vi "Autonomous Independent.vi"   [LabVIEW 2015]
doc: "This VI is called when autonomous begins, and will automatically be terminated when autonomous ends. You can carry out timed or sensor driven robot movement independently without needing to return to the caller."
uses:
  <vilib>/Rock Robotics/WPI/Utilities/WPI_GetSetVariantRefNum.vi
  <vilib>/Rock Robotics/Network Tables/NT Read String.vi
  <vilib>/Rock Robotics/Network Tables/NT Read Number.vi
  <vilib>/Rock Robotics/Network Tables/NT Read Boolean.vi
  <vilib>/Rock Robotics/Network Tables/NT Write Numeric Array.vi
panel:
  # "Be sure to right-click and choose Data Operations>>Make Current Value default if you want to save the array values with the VI"
types:
  T1 = typedef "WPI_JoystickDevRef.ctl" = cluster{"Device":T2}
  T2 = typedef "WPI_JoystickDeviceEnum.ctl" = enum16{"USB 0", "USB 1", "USB 2", "USB 3", "USB 4", "USB 5"}
  T3 = typedef "WPI_EncoderDevRef.ctl" = cluster{"DevStatus":errorcluster, "EncoderIndex":T4, "CounterIndex":T5, "DistancePerCount":dbl, "Decoding Type":T6}
  T4 = typedef "FPGA_EncoderIdx.ctl" = enum8{"Enc 0", "Enc 1", "Enc 2", "Enc 3", "Enc 4", "Enc 5", "Enc 6", "Enc 7", "Invalid"}
  T5 = typedef "FPGA_CounterCtrSystemIndex.ctl" = enum8{"Ctr 0", "Ctr 1", "Ctr 2", "Ctr 3", "Ctr 4", "Ctr 5", "Ctr 6", "Ctr 7", "Invalid"}
  T6 = typedef "WPI_EncoderType.ctl" = enum16{"1x", "2x", "4x"}
  T7 = typedef "WPI_GyroDevRef.ctl" = cluster{"DevStatus":errorcluster, "Analog Channel":T8, "Offset":dbl, "Gain (VoltsPerDegree/Second)":dbl, "Gyro Type":enum16{"Analog", "XRS450"}, "Handle":i32, "SPI Bus":T9, "Device Found":bool, "Sample Rate":dbl, "Calibrate On Open":bool}
  T8 = typedef "FPGA_AIChannel.ctl" = enum8{"AI 0", "AI 1", "AI 2", "AI 3", "AI MXP 0", "AI MXP 1", "AI MXP 2", "AI MXP 3", "Invalid"}
  T9 = typedef "spi_bus.ctl" = enum16{"SPI On-Board, CS0", "SPI On-Board, CS1", "SPI On-Board, CS2", "SPI On-Board, CS3", "SPI MXP", "Invalid"}
  T10 = typedef "WPI_RobotDriveDevRef.ctl" = cluster{"DevStatus":errorcluster, "Motors[]":T11[], "Square Inputs":bool, "Max Output":dbl}
  T11 = typedef "WPI_MotorControlDeviceRef.ctl" = cluster{"DeviceStatus":errorcluster, "Type":T12, "PWM":cluster{"PWM Channel":T13, "DeadBand":T14}, "CAN":cluster{"Device Number":u8, "Control Mode":T15, "Semaphore":T16, "Max Vout":dbl, "TalonSRX Control Mode":T17}, "Invert":bool}
  T12 = typedef "WPI_MotorControlType.ctl" = enum16{"PWM", "CAN", "CANTalonSRX"}
  T13 = typedef "FPGA_DIOPWMChannel.ctl" = enum8{"PWM 0", "PWM 1", "PWM 2", "PWM 3", "PWM 4", "PWM 5", "PWM 6", "PWM 7", "PWM 8", "PWM 9", "PWM MXP 0", "PWM MXP 1", "PWM MXP 2", "PWM MXP 3", "PWM MXP 4", "PWM MXP 5", "PWM MXP 6", "PWM MXP 7", "PWM MXP 8", "PWM MXP 9", "Invalid"}
  T14 = typedef "WPI_PWMDeadband.ctl" = cluster{"Name":string, "maxPositivePwm":i32, "minPositivePwm":i32, "centerPwm":i32, "maxNegativePwm":i32, "minNegativePwm":i32, "angularRange":u16}
  T15 = typedef "WPI_CANJaguar_ControlMode.ctl" = enum8{"Percent VBus", "Current", "Speed", "Position", "Voltage"}
  T16 = typedef "Semaphore RefNum" = refnum<k1>
  T17 = typedef "WPI_CANTalonSRX_APIControlMode.ctl" = enum8{"Percent VBus", "Speed", "Position", "Slave", "Unchanged / Invalid", "Voltage Compensation", "Current", "Motion Profile"}
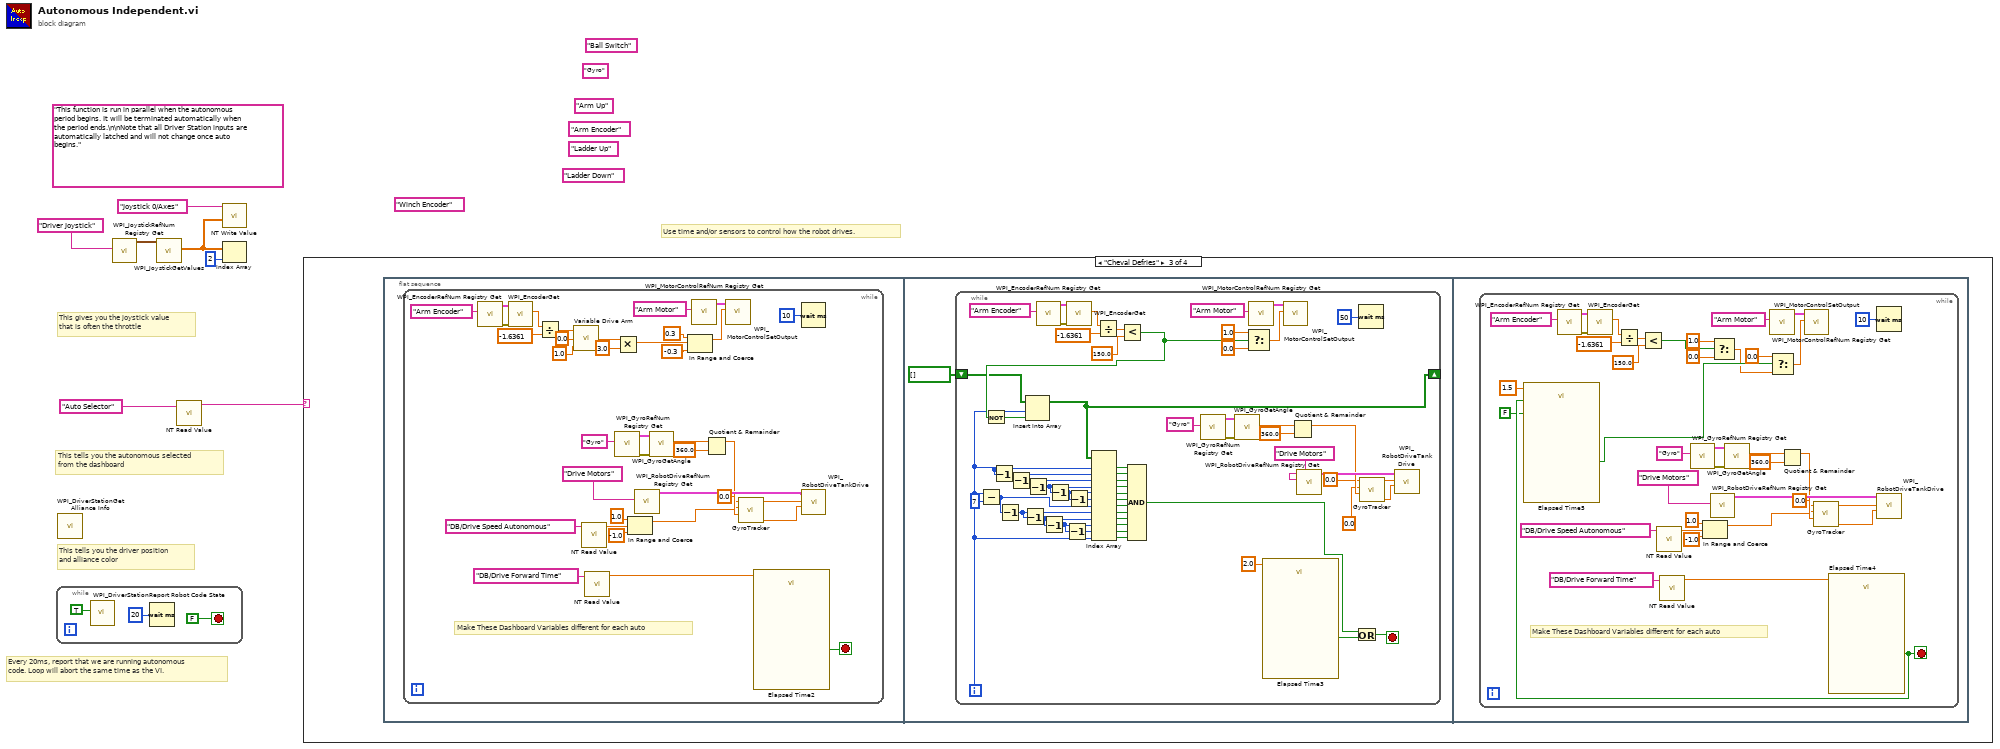
[diagram p0: block diagram]
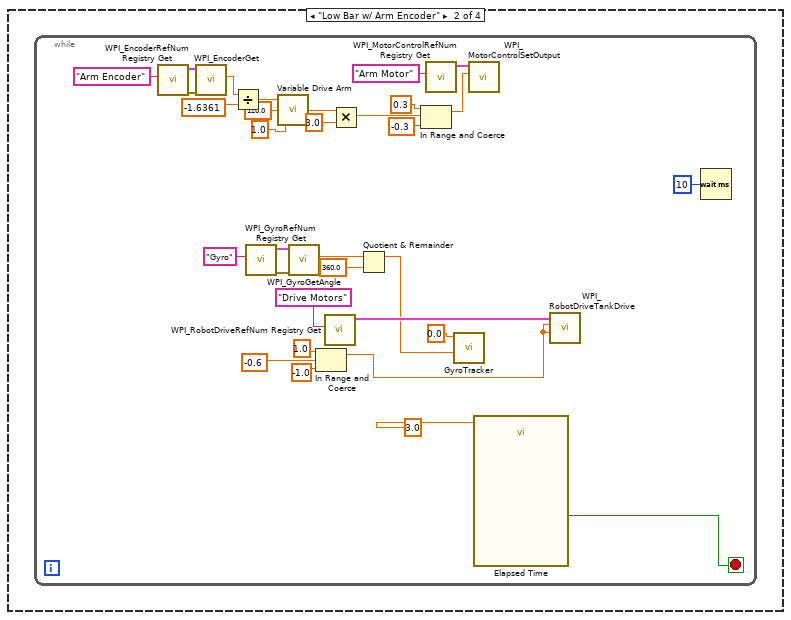
[diagram p3: hidden frame]
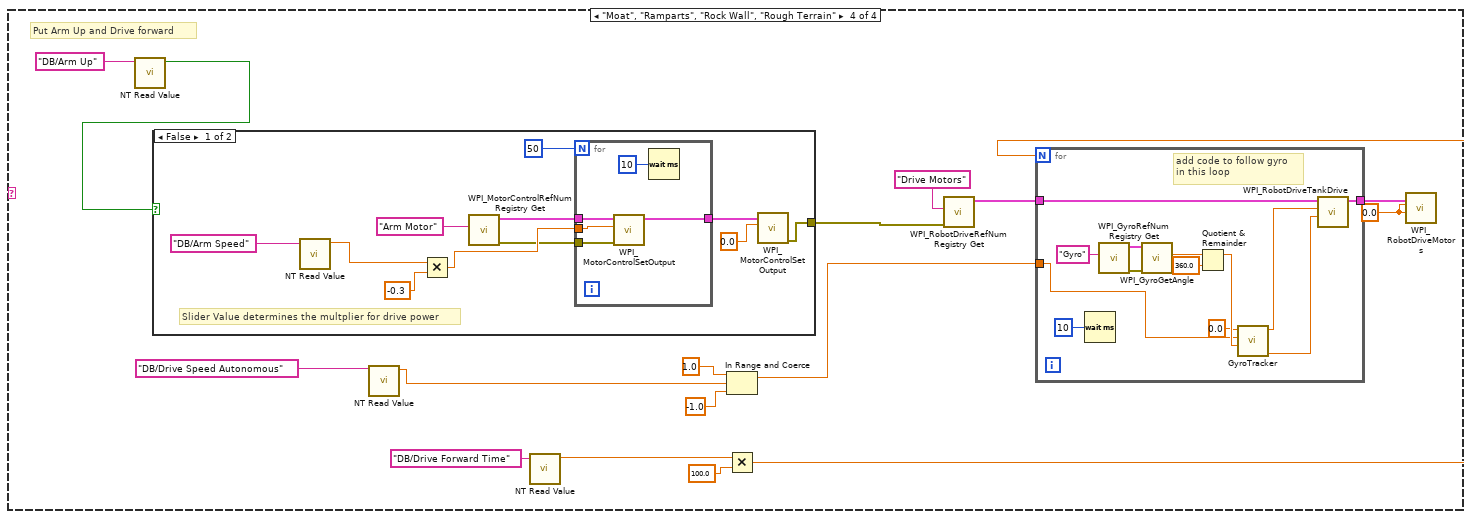
[diagram p4: hidden frame]
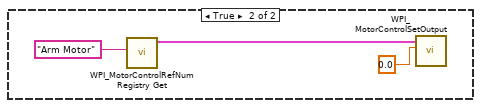
[diagram p5: hidden frame]
diagram:
  (unwired) "Arm Up" ("refnum name")
  (unwired) "Winch Encoder" ("refnum name")
  (unwired) "Ladder Down" ("refnum name")
  (unwired) "Ladder Up" ("refnum name")
  (unwired) "Arm Encoder" ("refnum name")
  (unwired) "Ball Switch" ("refnum name")
  (unwired) "Gyro" ("refnum name")
  (unwired) "This function is run in parallel when the autonomous period begins. It will be terminated automatically when the period ends.\n\nNote that all Driver Station inputs are automatically latched and will not change once auto begins."
  # "This tells you the autonomous selected\nfrom the dashboard"
  # "Every 20ms, report that we are running autonomous\ncode. Loop will abort the same time as the VI."
  # "This gives you the joystick value\nthat is often the throttle"
  # "Use time and/or sensors to control how the robot drives."
  # "This tells you the driver position\nand alliance color"
  n1 = while {
    stop <- FALSE stop-if-true
    n2 = call <vilib>:"WPI_DriverStationReport Robot Code State.vi"("Autonomous"=TRUE) -> ()  [unwired: 10 in, 1 out]
    n3 = Wait (ms)(milliseconds to wait=u32 20) -> ()  [unwired: 1 out]
  }
  n4 = call <vilib>:"WPI_DriverStationGet Alliance Info.vi"() -> ()  [unwired: 12 out]
  n5 = call <vilib>:"WPI_JoystickRefNum Registry Get.vi"("refnum name"="Driver Joystick") -> ("JoystickDevRef"=w6:T1)  [unwired: 1 in, 9 out]
  n6 = call <vilib>:"WPI_JoystickGetValues.vi"("JoystickDevRef"=w6) -> ("Axes"=w2:dbl[])  [unwired: 6 in, 4 out]
  n7 = call-poly <vilib>:"NT Read Value.vi"("Name"="Auto Selector") -> ("String"=w3:string)  [unwired: 9 in, 1 out]
  n8 = call-poly <vilib>:"NT Write Value.vi"("Numeric Array"=w2, "Name"="Joystick 0/Axes") -> ()  [unwired: 9 in, 1 out]
  n9 = Index Array(array=w2, index=2) -> ()  [unwired: 1 out]
  n10 = case shown="\"Cheval Defries\"" w3 {
    frame Default {
      # "You can put your main auto here, or you can right-click on the case and make any\nother frame be the default case."
      # "This is the frame that will execute if no selection is made, or if it is not recognized"
    }
    frame "Low Bar w/ Arm Encoder" {
      n11 = while {
        stop <- w42 stop-if-true
        n12 = call <vilib>:"WPI_EncoderRefNum Registry Get.vi"("refnum name"="Arm Encoder") -> ("error out"=w35:errorcluster, "EncoderDevRef"=w36:T3)  [unwired: 9 in]
        n13 = call <vilib>:"WPI_EncoderGet.vi"("error in (no error)"=w35, "EncoderDevRef"=w36) -> ("Distance"=w37:dbl)  [unwired: 4 in, 5 out]
        n14 = Divide(x=w37, y=-1.6361 ("Arm Calibration")) -> (x/y=w34:dbl)
        n15 = call <vilib>:"WPI_GyroRefNum Registry Get.vi"("refnum name"="Gyro") -> ("error out"=w16:errorcluster, "GyroDevRef"=w17:T7)  [unwired: 9 in]
        n16 = call "Variable Drive Arm.vi"("Max Speed"=1.0, "Wanted Angle"=120.0, "Encoder"=w34) -> ("Motor Controller"=w27:dbl)
        n17 = call <vilib>:"WPI_GyroGetAngle.vi"("error in"=w16, "GyroDevRef"=w17) -> ("Angle"=w19:dbl)  [unwired: 5 in, 4 out]
        n18 = In Range and Coerce(upper limit=1.0, x=-0.6, lower limit=-1.0) -> (coerced(x)=w13:dbl)  [unwired: 1 out]
        n19 = call <vilib>:"WPI_RobotDriveRefNum Registry Get.vi"("refnum name"="Drive Motors") -> ("RobotDriveDevRef"=w24:T10)  [unwired: 1 in, 9 out]
        n20 = Multiply(x=w27, y=3.0) -> (x*y=w25:dbl)
        n21 = Quotient & Remainder(x=w19, y=360.0) -> (x-y*floor(x/y)=w15:dbl)  [unwired: 1 out]
        n22 = In Range and Coerce(upper limit=0.3, x=w25, lower limit=-0.3) -> (coerced(x)=w30:dbl)  [unwired: 1 out]
        n23 = call <vilib>:"WPI_MotorControlRefNum Registry Get.vi"("refnum name"="Arm Motor") -> ("MotorControlDevRef"=w31:T11)  [unwired: 9 in, 1 out]
        n24 = call "GyroTracker.vi"("Gyro Angle"=w15, "Target Direction (degrees)"=0.0) -> ()  [unwired: 8 in, 2 out]
        n25 = call <vilib>:"WPI_MotorControlSetOutput.vi"("Output"=w30, "MotorControlDevRef"=w31) -> ()  [unwired: 7 in, 3 out]
        n26 = call "Elapsed Time"("Time Target (s)"=3.0) -> ("Time has Elapsed"=w42:bool)  [unwired: 11 in, 7 out]
        n27 = call <vilib>:"WPI_RobotDriveTankDrive.vi"("Right axis value"=w13, "Left axis value"=w13, "RobotDriveDevRef"=w24) -> ()  [unwired: 6 in, 3 out]
        n28 = Wait (ms)(milliseconds to wait=u32 10) -> ()  [unwired: 1 out]
      }
    }
    frame "Cheval Defries" {
      n29 = flat-sequence {
        frame #0 {
          n30 = while {
            stop <- w78 stop-if-true
            # "Make These Dashboard Variables different for each auto"
            n31 = call <vilib>:"WPI_EncoderRefNum Registry Get.vi"("refnum name"="Arm Encoder") -> ("error out"=w71:errorcluster, "EncoderDevRef"=w72:T3)  [unwired: 9 in]
            n32 = call <vilib>:"WPI_EncoderGet.vi"("error in (no error)"=w71, "EncoderDevRef"=w72) -> ("Distance"=w73:dbl)  [unwired: 4 in, 5 out]
            n33 = Divide(x=w73, y=-1.6361 ("Arm Calibration")) -> (x/y=w70:dbl)
            n34 = call "Variable Drive Arm.vi"("Max Speed"=1.0, "Wanted Angle"=0.0, "Encoder"=w70) -> ("Motor Controller"=w63:dbl)
            n35 = call-poly <vilib>:"NT Read Value.vi"("Name"="DB/Drive Speed Autonomous") -> ("Numeric"=w57:dbl)  [unwired: 9 in, 1 out]
            n36 = call-poly <vilib>:"NT Read Value.vi"("Name"="DB/Drive Forward Time") -> ("Numeric"=w55:dbl)  [unwired: 9 in, 1 out]
            n37 = call <vilib>:"WPI_GyroRefNum Registry Get.vi"("refnum name"="Gyro") -> ("error out"=w46:errorcluster, "GyroDevRef"=w47:T7)  [unwired: 9 in]
            n38 = Multiply(x=w63, y=3.0) -> (x*y=w61:dbl)
            n39 = In Range and Coerce(upper limit=1.0, x=w57, lower limit=-1.0) -> (coerced(x)=w43:dbl)  [unwired: 1 out]
            n40 = call <vilib>:"WPI_RobotDriveRefNum Registry Get.vi"("refnum name"="Drive Motors") -> ("RobotDriveDevRef"=w53:T10)  [unwired: 1 in, 9 out]
            n41 = call <vilib>:"WPI_GyroGetAngle.vi"("error in"=w46, "GyroDevRef"=w47) -> ("Angle"=w49:dbl)  [unwired: 5 in, 4 out]
            n42 = In Range and Coerce(upper limit=0.3, x=w61, lower limit=-0.3) -> (coerced(x)=w66:dbl)  [unwired: 1 out]
            n43 = call <vilib>:"WPI_MotorControlRefNum Registry Get.vi"("refnum name"="Arm Motor") -> ("MotorControlDevRef"=w67:T11)  [unwired: 9 in, 1 out]
            n44 = Quotient & Remainder(x=w49, y=360.0) -> (x-y*floor(x/y)=w45:dbl)  [unwired: 1 out]
            n45 = call <vilib>:"WPI_MotorControlSetOutput.vi"("Output"=w66, "MotorControlDevRef"=w67) -> ()  [unwired: 7 in, 3 out]
            n46 = call "GyroTracker.vi"("Gyro Angle"=w45, "Target Speed"=w43, "Target Direction (degrees)"=0.0) -> ("Right Wheel Speed"=w51:dbl, "Left Wheel Speed"=w52:dbl)  [unwired: 7 in]
            n47 = call "Elapsed Time2"("Time Target (s)"=w55) -> ("Time has Elapsed"=w78:bool)  [unwired: 11 in, 7 out]
            n48 = Wait (ms)(milliseconds to wait=u32 10) -> ()  [unwired: 1 out]
            n49 = call <vilib>:"WPI_RobotDriveTankDrive.vi"("Right axis value"=w51, "Left axis value"=w52, "RobotDriveDevRef"=w53) -> ()  [unwired: 6 in, 3 out]
          }
        }
        frame #1 {
          n50 = while {
            shift-right: [w84] -> _
            shift-left: bool[] [] -> [w85]
            i -> [w83]
            stop <- w88 stop-if-true
            n51 = Subtract(x=w83, y=7) -> (x-y=w105:i32)
            n52 = Decrement(x=w83) -> (x-1=w108:i32)
            n53 = Decrement(x=w105) -> (x-1=w104:i32)
            n54 = Decrement(x=w108) -> (x-1=w110:i32)
            n55 = Decrement(x=w104) -> (x-1=w103:i32)
            n56 = Decrement(x=w110) -> (x-1=w112:i32)
            n57 = call <vilib>:"WPI_EncoderRefNum Registry Get.vi"("refnum name"="Arm Encoder") -> ("error out"=w118:errorcluster, "EncoderDevRef"=w119:T3)  [unwired: 9 in]
            n58 = Decrement(x=w103) -> (x-1=w101:i32)
            n59 = Decrement(x=w112) -> (x-1=w109:i32)
            n60 = Decrement(x=w101) -> (x-1=w102:i32)
            n61 = call <vilib>:"WPI_EncoderGet.vi"("error in (no error)"=w118, "EncoderDevRef"=w119) -> ("Distance"=w120:dbl)  [unwired: 4 in, 5 out]
            n62 = Decrement(x=w109) -> (x-1=w111:i32)
            n63 = Divide(x=w120, y=-1.6361 ("Arm Calibration")) -> (x/y=w113:dbl)
            n64 = Less?(x=w113, y=150.0) -> (x < y?=w86:bool)
            n65 = Not(x=w86) -> (.not. x?=w80:bool)
            n66 = Insert Into Array(array=w85, index=w83, new element=w80) -> (w84:bool[])
            n67 = Index Array(array=w84, index #1=w83, index #2=w108, index #3=w110, index #4=w112, index #5=w109, index #6=w111, index #7=w105, index #8=w104, index #9=w103, index #10=w101, index #11=w102, index #12=w83) -> (element #1=w100:bool, element #2=w99:bool, element #3=w98:bool, element #4=w97:bool, element #5=w96:bool, element #6=w95:bool, element #7=w94:bool, element #8=w93:bool, element #9=w92:bool, element #10=w91:bool, element #11=w90:bool, element #12=w82:bool)
            n68 = Compound Arithmetic op=AND(w100, w99, w98, w97, w96, w95, w94, w93, w92, w91, w90, w82) -> (w81:bool)
            n69 = call <vilib>:"WPI_GyroRefNum Registry Get.vi"("refnum name"="Gyro") -> ("error out"=w126:errorcluster, "GyroDevRef"=w127:T7)  [unwired: 9 in]
            n70 = call <vilib>:"WPI_GyroGetAngle.vi"("error in"=w126, "GyroDevRef"=w127) -> ("Angle"=w129:dbl)  [unwired: 5 in, 4 out]
            n71 = Select(t=1.0, s=w86, f=0.0) -> (s? t:f=w116:dbl)
            n72 = call <vilib>:"WPI_MotorControlRefNum Registry Get.vi"("refnum name"="Arm Motor") -> ("MotorControlDevRef"=w135:T11)  [unwired: 9 in, 1 out]
            n73 = call "Elapsed Time3"("Time Target (s)"=2.0) -> ("Time has Elapsed"=w89:bool)  [unwired: 11 in, 7 out]
            n74 = call <vilib>:"WPI_MotorControlSetOutput.vi"("Output"=w116, "MotorControlDevRef"=w135) -> ()  [unwired: 7 in, 3 out]
            n75 = Quotient & Remainder(x=w129, y=360.0) -> (x-y*floor(x/y)=w125:dbl)  [unwired: 1 out]
            n76 = call <vilib>:"WPI_RobotDriveRefNum Registry Get.vi"("refnum name"="Drive Motors") -> ("RobotDriveDevRef"=w132:T10)  [unwired: 1 in, 9 out]
            n77 = Or(x=w81, y=w89) -> (x .or. y?=w88:bool)
            n78 = Wait (ms)(milliseconds to wait=u32 50) -> ()  [unwired: 1 out]
            n79 = call "GyroTracker.vi"("Gyro Angle"=w125, "Target Speed"=0.0, "Target Direction (degrees)"=0.0) -> ("Right Wheel Speed"=w107:dbl, "Left Wheel Speed"=w131:dbl)  [unwired: 7 in]
            n80 = call <vilib>:"WPI_RobotDriveTankDrive.vi"("Right axis value"=w107, "Left axis value"=w131, "RobotDriveDevRef"=w132) -> ()  [unwired: 6 in, 3 out]
          }
        }
        frame #2 {
          n81 = while {
            stop <- w142 stop-if-true
            # "Make These Dashboard Variables different for each auto"
            n82 = call <vilib>:"WPI_EncoderRefNum Registry Get.vi"("refnum name"="Arm Encoder") -> ("error out"=w149:errorcluster, "EncoderDevRef"=w150:T3)  [unwired: 9 in]
            n83 = call <vilib>:"WPI_EncoderGet.vi"("error in (no error)"=w149, "EncoderDevRef"=w150) -> ("Distance"=w151:dbl)  [unwired: 4 in, 5 out]
            n84 = Divide(x=w151, y=-1.6361 ("Arm Calibration")) -> (x/y=w145:dbl)
            n85 = Less?(x=w145, y=150.0) -> (x < y?=w144:bool)
            n86 = call-poly <vilib>:"NT Read Value.vi"("Name"="DB/Drive Speed Autonomous") -> ("Numeric"=w170:dbl)  [unwired: 9 in, 1 out]
            n87 = call-poly <vilib>:"NT Read Value.vi"("Name"="DB/Drive Forward Time") -> ("Numeric"=w168:dbl)  [unwired: 9 in, 1 out]
            n88 = call <vilib>:"WPI_GyroRefNum Registry Get.vi"("refnum name"="Gyro") -> ("error out"=w159:errorcluster, "GyroDevRef"=w160:T7)  [unwired: 9 in]
            n89 = In Range and Coerce(upper limit=1.0, x=w170, lower limit=-1.0) -> (coerced(x)=w156:dbl)  [unwired: 1 out]
            n90 = call <vilib>:"WPI_RobotDriveRefNum Registry Get.vi"("refnum name"="Drive Motors") -> ("RobotDriveDevRef"=w166:T10)  [unwired: 1 in, 9 out]
            n91 = Select(t=1.0, s=w144, f=0.0) -> (s? t:f=w137:dbl)
            n92 = call <vilib>:"WPI_GyroGetAngle.vi"("error in"=w159, "GyroDevRef"=w160) -> ("Angle"=w162:dbl)  [unwired: 5 in, 4 out]
            n93 = call <vilib>:"WPI_MotorControlRefNum Registry Get.vi"("refnum name"="Arm Motor") -> ("MotorControlDevRef"=w154:T11)  [unwired: 9 in, 1 out]
            n94 = Quotient & Remainder(x=w162, y=360.0) -> (x-y*floor(x/y)=w158:dbl)  [unwired: 1 out]
            n95 = call "GyroTracker.vi"("Gyro Angle"=w158, "Target Speed"=w156, "Target Direction (degrees)"=0.0) -> ("Right Wheel Speed"=w164:dbl, "Left Wheel Speed"=w165:dbl)  [unwired: 7 in]
            n96 = call "Elapsed Time4"("Time Target (s)"=w168) -> ("Time has Elapsed"=w142:bool)  [unwired: 11 in, 7 out]
            n97 = call "Elapsed Time5"("Time Target (s)"=1.5, "Reset"=w142, "Auto Reset"=FALSE) -> ("Time has Elapsed"=w139:bool)  [unwired: 9 in, 7 out]
            n98 = Select(t=0.0, s=w139, f=w137) -> (s? t:f=w140:dbl)
            n99 = call <vilib>:"WPI_MotorControlSetOutput.vi"("Output"=w140, "MotorControlDevRef"=w154) -> ()  [unwired: 7 in, 3 out]
            n100 = Wait (ms)(milliseconds to wait=u32 10) -> ()  [unwired: 1 out]
            n101 = call <vilib>:"WPI_RobotDriveTankDrive.vi"("Right axis value"=w164, "Left axis value"=w165, "RobotDriveDevRef"=w166) -> ()  [unwired: 6 in, 3 out]
          }
        }
      }
    }
    frame "Moat", "Ramparts", "Rock Wall", "Rough Terrain" {
      w187 = 0.0 ("Y axis value")
      # "Put Arm Up and Drive forward"
      n102 = call-poly <vilib>:"NT Read Value.vi"("Name"="DB/Arm Up") -> ("Boolean"=w180:bool)  [unwired: 9 in, 1 out]
      n103 = case shown="False" w180 {
        tunnel: [w191 _] -> w181
        frame False {
          # "Slider Value determines the multplier for drive power"
          n104 = call-poly <vilib>:"NT Read Value.vi"("Name"="DB/Arm Speed") -> ("Numeric"=w196:dbl)  [unwired: 9 in, 1 out]
          n105 = Multiply(x=w196, y=-0.3) -> (x*y=w201:dbl)
          n106 = call <vilib>:"WPI_MotorControlRefNum Registry Get.vi"("refnum name"="Arm Motor") -> ("error out"=w200:errorcluster, "MotorControlDevRef"=w199:T11)  [unwired: 9 in]
          n107 = for {
            N: 50 -> [_]
            tunnel: w199 -> [w205]
            tunnel: w200 -> [w204]
            tunnel: w201 -> [w203]
            tunnel: [w202] -> w192
            n108 = call <vilib>:"WPI_MotorControlSetOutput.vi"("error in (no error)"=w204, "Output"=w203, "MotorControlDevRef"=w205) -> ("MotorControlDevRef"=w202:T11)  [unwired: 6 in, 2 out]
            n109 = Wait (ms)(milliseconds to wait=u32 10) -> ()  [unwired: 1 out]
          }
          n110 = call <vilib>:"WPI_MotorControlSetOutput.vi"("Output"=0.0, "MotorControlDevRef"=w192) -> ("error out"=w191:errorcluster)  [unwired: 7 in, 2 out]
        }
        frame True {
          n111 = call <vilib>:"WPI_MotorControlRefNum Registry Get.vi"("refnum name"="Arm Motor") -> ("MotorControlDevRef"=w208:T11)  [unwired: 9 in, 1 out]
          n112 = call <vilib>:"WPI_MotorControlSetOutput.vi"("Output"=0.0, "MotorControlDevRef"=w208) -> ()  [unwired: 7 in, 3 out]
        }
      }
      n113 = call-poly <vilib>:"NT Read Value.vi"("Name"="DB/Drive Speed Autonomous") -> ("Numeric"=w185:dbl)  [unwired: 9 in, 1 out]
      n114 = call-poly <vilib>:"NT Read Value.vi"("Name"="DB/Drive Forward Time") -> ("Numeric"=w177:dbl)  [unwired: 9 in, 1 out]
      n115 = In Range and Coerce(upper limit=1.0, x=w185, lower limit=-1.0) -> (coerced(x)=w179:dbl)  [unwired: 1 out]
      n116 = Multiply(x=w177, y=100.0) -> (x*y=w175:dbl)
      n117 = call <vilib>:"WPI_RobotDriveRefNum Registry Get.vi"("error in (no error)"=w181, "refnum name"="Drive Motors") -> ("RobotDriveDevRef"=w189:T10)  [unwired: 9 out]
      n118 = for {
        N: w175 -> [_]
        tunnel: w189 -> [w212]
        tunnel: w179 -> [w210]
        tunnel: [w211] -> w188
        # "add code to follow gyro\nin this loop"
        n119 = Wait (ms)(milliseconds to wait=u32 10) -> ()  [unwired: 1 out]
        n120 = call <vilib>:"WPI_GyroRefNum Registry Get.vi"("refnum name"="Gyro") -> ("error out"=w215:errorcluster, "GyroDevRef"=w216:T7)  [unwired: 9 in]
        n121 = call <vilib>:"WPI_GyroGetAngle.vi"("error in"=w215, "GyroDevRef"=w216) -> ("Angle"=w218:dbl)  [unwired: 5 in, 4 out]
        n122 = Quotient & Remainder(x=w218, y=360.0) -> (x-y*floor(x/y)=w214:dbl)  [unwired: 1 out]
        n123 = call "GyroTracker.vi"("Gyro Angle"=w214, "Target Speed"=w210, "Target Direction (degrees)"=0.0) -> ("Right Wheel Speed"=w220:dbl, "Left Wheel Speed"=w221:dbl)  [unwired: 7 in]
        n124 = call <vilib>:"WPI_RobotDriveTankDrive.vi"("Right axis value"=w220, "Left axis value"=w221, "RobotDriveDevRef"=w212) -> ("RobotDriveDevRef"=w211:T10)  [unwired: 6 in, 2 out]
      }
      n125 = call <vilib>:"WPI_RobotDriveMotors.vi"("RightSpeed"=w187, "LeftSpeed"=w187, "RobotDriveDevRef"=w188) -> ()  [unwired: 6 in, 3 out]
    }
  }
